vi "Send Handle and Broadcast Event.vi"(7 "Priority":T1=enum."Normal" caption="Message Priority (Normal)", 8 "error in (no error)":errorcluster, 9 "Event Data":refnum<class "Event.lvclass">, 10 "View Enqueuer":refnum<class "Message Enqueuer.lvclass">, 11 "Message Enqueuer in":refnum<class "Message Enqueuer.lvclass">) -> (0 "error out":errorcluster, 3 "Message Enqueuer out":refnum<class "Message Enqueuer.lvclass">)   [LabVIEW 2023, in "MVC Actors.lvlib" / "Handle and Broadcast Event Msg.lvclass"]
doc: "Sends the <b>MVC Actors.lvlib:Handle and Broadcast Event Msg.lvclass</b> message.\n\nThis message will call <b>Handle and Broadcast Event.vi</b> on the <b>MVC Actors.lvlib:Controller.lvclass</b> actor.\n\n<b>Handle and Broadcast Event.vi Description</b>\nThis method generates/fires the Event wired to the input triggered by a View. Firing an event originating form a View looks up all actors, but the originating View, who registered to listen to this Event and sends to them this Event on a Zero Coupling based message defined during registration. Errors on broadcasting the event i.e. enqueuer of the registrant not existing, are ignored.\n\n<b>IMPORTANT</b> - Only call this method directly (not through the corresponding message) within actor method calls of your Controller Actor. From helper loops send to self the corresponding message by means of its send method. This is to make sure your controller acts all the currently registered listeners."
uses:
  Handle and Broadcast Event Msg.lvclass
  Handle and Broadcast Event Msg.lvclass/Handle and Broadcast Event Msg.ctl
  <vilib>/ActorFramework/Message Enqueuer/Message Enqueuer.lvclass
  C:/Program Files/National Instruments/LabVIEW 2023/vi.lib/ActorFramework/Message/Message.lvclass
  C:/Projects/Shared Libraries/Event Actors/Controller Messages/Handle and Broadcast Event Msg/Handle and Broadcast Event Msg.lvclass
  <vilib>/ActorFramework/Message Enqueuer/Message Priority.ctl
  Event/Event.lvclass
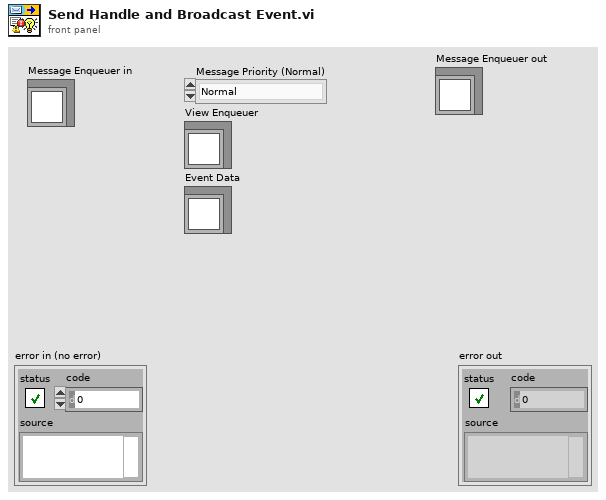
[diagram p1: front panel]
types:
  T1 = typedef "Actor Framework.lvlib/Message Enqueuer.lvclass/Message Priority.ctl" = enum16{"Low", "Normal", "High"}
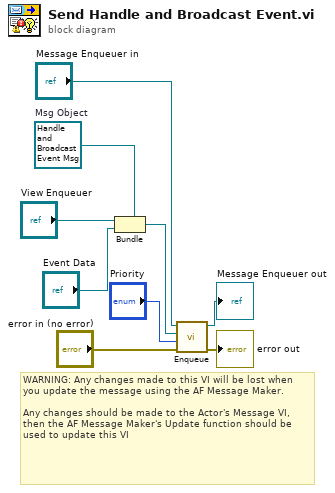
[diagram p0: block diagram]
diagram:
  w7 = refnum<class "Handle and Broadcast Event Msg.lvclass"> refnum  # Msg Object
  # "WARNING: Any changes made to this VI will be lost when you update the message using the AF Message Maker.\n\nAny changes should be made to the Actor's Message VI, then the AF Message Maker's Update function should be used to update this VI"
  n1 = Bundle(cluster=w7, "View Enqueuer", "Event Data") -> (w2:refnum<class "Handle and Broadcast Event Msg.lvclass">)
  n2 = call <vilib>:"Enqueue.vi"("error in (no error)"="error in (no error)", "Message Priority (Normal)"="Priority", "Message"=w2, "Message Enqueuer in"="Message Enqueuer in") -> ("error out"=→"error out":errorcluster, "Message Enqueuer out"=→"Message Enqueuer out":refnum<class "Message Enqueuer.lvclass">)  [unwired: 6 in]
